vi "Update_Time.vi"(0 "Total Time Elapsed In":dbl, 1 "Total Time":dbl, 2 "Current Event Time":dbl, 3 "Iteration":i32, 4 "Delta Time (s)":dbl) -> (5 "Total Time Elapsed Out":dbl, 6 "End":bool, 7 "Output Times":T1)   [LabVIEW 2011]
doc: "This VI takes a number of time-related inputs and uses them to calculate an output cluster with information pertaining to the time remaining in the growth sequence."
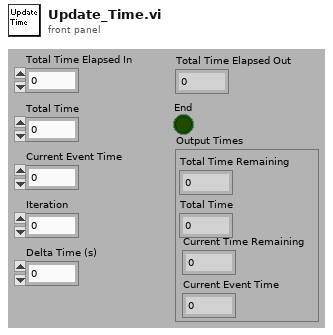
[diagram p1: front panel]
types:
  T1 = cluster{"Total Time Remaining":dbl, "Total Time":dbl, "Current Time Remaining":dbl, "Current Event Time":dbl}
  T2 = cluster{dbl, "Total Time":dbl, dbl, "Current Event Time":dbl}
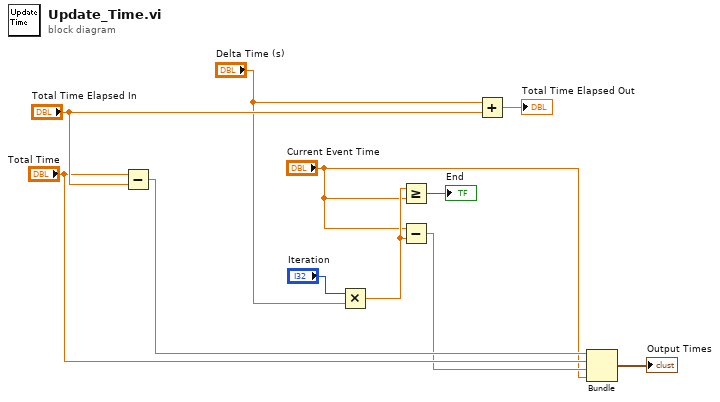
[diagram p0: block diagram]
diagram:
  n1 = Subtract(x="Total Time", y="Total Time Elapsed In") -> (x-y=w6:dbl)
  n2 = Multiply(x="Iteration", y="Delta Time (s)") -> (x*y=w9:dbl)
  n3 = Greater Or Equal?(x=w9, y="Current Event Time") -> (x >= y?=→"End":bool)
  n4 = Subtract(x="Current Event Time", y=w9) -> (x-y=w4:dbl)
  n5 = Add(x="Delta Time (s)", y="Total Time Elapsed In") -> (x+y=→"Total Time Elapsed Out":dbl)
  n6 = Bundle(w6, "Total Time"="Total Time", w4, "Current Event Time"="Current Event Time") -> (→"Output Times":T2)  [unwired: 1 out]
